vi "Calculate moves.vi"(7 "Position":refnum<class "Position.lvclass">, 8 "error in (no error)":errorcluster, 10 "Source":T1={"File"=enum."d", "Rank"=enum."4"}, 11 "Rook in":refnum<class "Rook.lvclass">) -> (0 "error out":errorcluster, 2 "Moves":refnum<class "Move.lvclass">[](array[class]), 3 "Rook out":refnum<class "Rook.lvclass">)   [LabVIEW 2016, in "Chesslib.lvlib" / "Rook.lvclass"]
uses:
  Rook.lvclass
  C:/Users/GRTaggJ/Documents/Projects/chesslib/Pieces/Runner/Runner.lvclass
  Moves/Move/Move.lvclass
  typedef/Square.ctl
  typedef/File.ctl
  typedef/Rank.ctl
  Position/Position.lvclass
  typedef/Direction.ctl
  Runner/Runner.lvclass
  Chesslib.lvlib
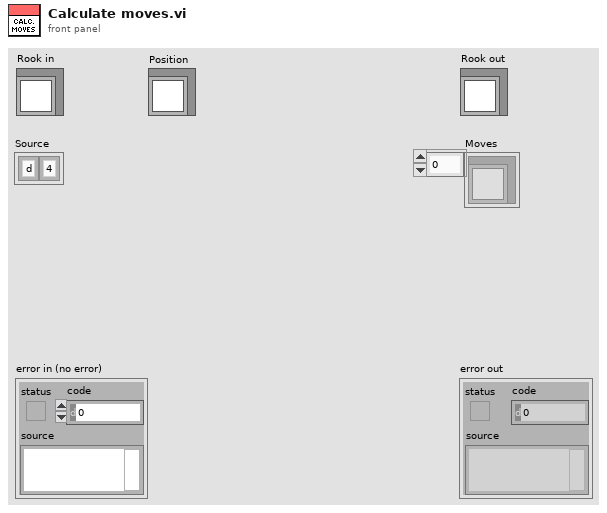
[diagram p1: front panel]
types:
  T1 = typedef "Chesslib.lvlib/Square.ctl" = cluster{"File":T2, "Rank":T3}
  T2 = typedef "Chesslib.lvlib/File.ctl" = enum8{"a", "b", "c", "d", "e", "f", "g", "h"}
  T3 = typedef "Chesslib.lvlib/Rank.ctl" = enum8{"1", "2", "3", "4", "5", "6", "7", "8"}
  T4 = typedef "Chesslib.lvlib/Direction.ctl" = enum16{"Straight", "Diagonal", "Both"}
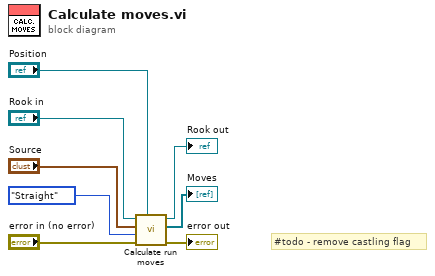
[diagram p0: block diagram]
diagram:
  # "#todo - remove castling flag"
  n1 = call "Calculate run moves.vi"("Position"="Position", "error in (no error)"="error in (no error)", "Direction"=Direction."Straight", "Source"="Source", "Runner in"="Rook in") -> ("error out"=→"error out":errorcluster, "Moves"=→"Moves":refnum<class "Move.lvclass">[], "Runner out"=→"Rook out":refnum<class "Rook.lvclass">)  [unwired: 4 in]
